vi "Write PID per ID.vi"(8 "error in (no error)":errorcluster, 10 "PID per ID":T1[](array[typedef]), 11 "Parameters in":refnum<class "Parameters.lvclass">) -> (0 "error out":errorcluster, 3 "Parameters out":refnum<class "Parameters.lvclass">)   [LabVIEW 2023, in "Parameters.lvclass"]
uses:
  Parameters.lvclass
  Controls/PIDParameters.ctl
  Parameters.lvclass/Parameters.ctl
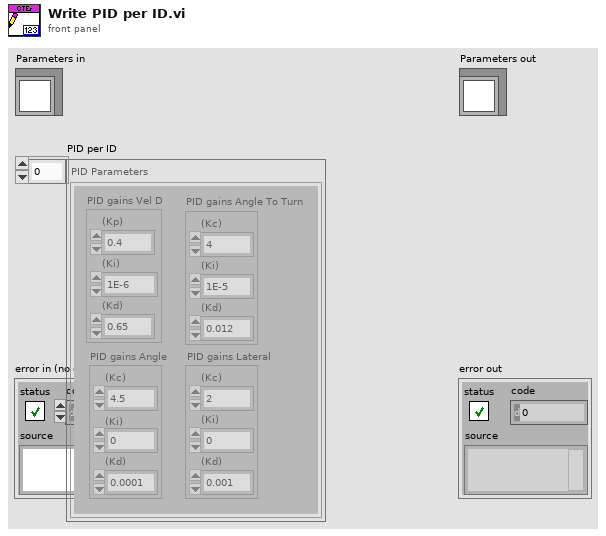
[diagram p1: front panel]
types:
  T1 = typedef "PIDParameters.ctl" = cluster{"PID gains Vel D":cluster{"(Kp)":dbl, "(Ki)":dbl, "(Kd)":dbl}, "PID gains Angle":cluster{"(Kc)":dbl, "(Ki)":dbl, "(Kd)":dbl}, "PID gains Angle To Turn":cluster{"(Kc)":dbl, "(Ki)":dbl, "(Kd)":dbl}, "PID gains Lateral":cluster{"(Kc)":dbl, "(Ki)":dbl, "(Kd)":dbl}}
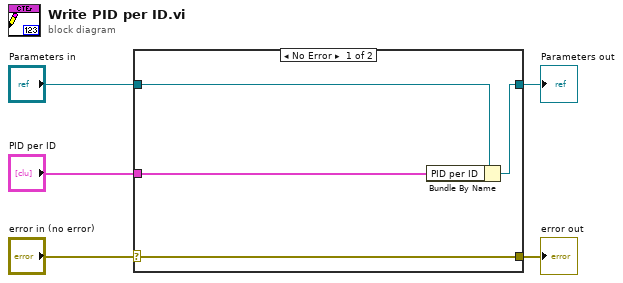
[diagram p0: block diagram]
diagram:
  n1 = case shown="No Error" "error in (no error)" {
    selector: "error in (no error)" -> [w9 w10]
    tunnel: [w9 w10] -> w4
    tunnel: [w7 w11] -> w2
    tunnel: "Parameters in" -> [w8 w11]
    tunnel: "PID per ID" -> [w6 _]
    frame No Error {
      n2 = Bundle By Name(cluster=w8, "PID per ID"=w6) -> (w7:refnum<class "Parameters.lvclass">)
    }
    frame Error {
    }
  }
  "error out" <- w4
  "Parameters out" <- w2
